vi "Grenzwerte SysLog.vi"(9 "Anlagen-Grenzwerte Anzeige":T1[](array[typedef]) {"Regler" items=["inaktiv", "aktiv"]; "Abschalt-Max" format="%#_5g"; "Abschalt-Min" format="%#_5g"; "Warn-Max" format="%#_5g"; "Warn-Min" format="%#_5g"; "Sollwert" format="%#_5g"}, 10 "Fehlermeldung":string[](array[string]), 11 "NewVal":T1[](array[typedef]) {"Regler" items=["inaktiv", "aktiv"]; "Abschalt-Max" format="%#_5g"; "Abschalt-Min" format="%#_5g"; "Warn-Max" format="%#_5g"; "Warn-Min" format="%#_5g"; "Sollwert" format="%#_5g"}) -> ()   [LabVIEW 2015, in "Anlagengrenzwerte.lvlib"]
uses:
  Anlagengrenzwerte.lvlib
  Anlagen-Parameter Anzeige.ctl
  Visualisierungs Elemente/Zahlen-Eingabefeld.ctl
  SysLog/SysLog Interface.ctl
  SysLog/SysLog.lvlib
panel:
  # "°C"
  # "°C"
  # "°C"
  # "°C"
  # "°C"
  # "°C"
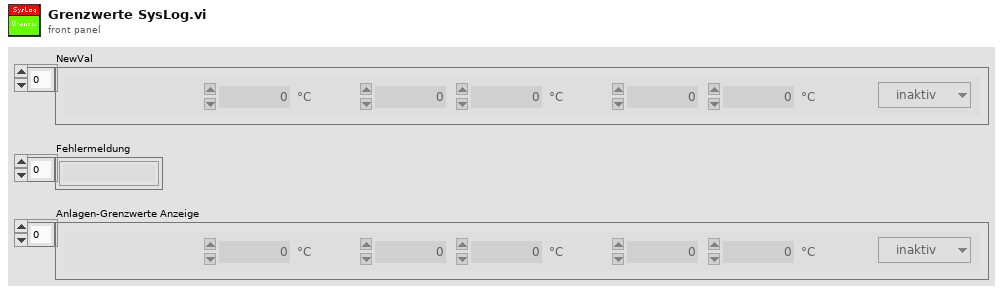
[diagram p1: front panel]
types:
  T1 = typedef "Anlagengrenzwerte.lvlib/Anlagen-Parameter Anzeige.ctl" = cluster{"Sollwert":T2, "Warn-Min":T2, "Warn-Max":T2, "Abschalt-Min":T2, "Abschalt-Max":T2, "Regler":u16}
  T2 = typedef "Zahlen-Eingabefeld.ctl" = sgl
  T3 = typedef "SysLog.lvlib/SysLog Interface.ctl" = cluster{"FehlermeldungsCode":i32, "ErfolgsmeldungsCode":i32, "ParameterListenString":string, "Anzeige":bool, "SysLogIcon":enum16{"OK", "Warnung", "Fehler"}, "intern":bool}
  T4 = cluster{"Sollwert":T2, "Warn-Min":T2, "Warn-Max":T2, "Abschalt-Min":T2, "Abschalt-Max":T2, "Regler":sgl}
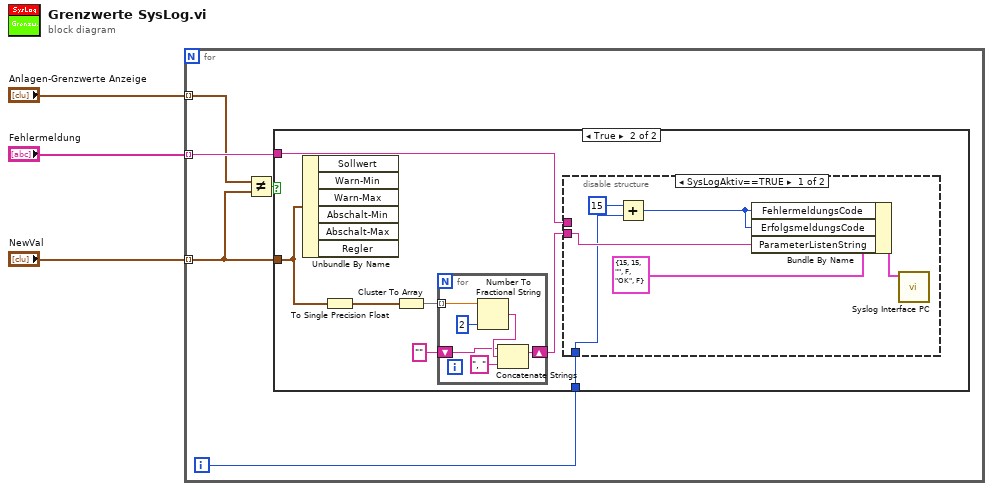
[diagram p0: block diagram]
diagram:
  n1 = for {
    tunnel: "NewVal" -> [w6] mode=indexing
    tunnel: "Anlagen-Grenzwerte Anzeige" -> [w7] mode=indexing
    tunnel: "Fehlermeldung" -> [w8] mode=indexing
    i -> [w4]
    n2 = Not Equal?(x=w7, y=w6) -> (x != y?=w5:bool)
    n3 = case shown="True" w5 {
      tunnel: w8 -> [_ w15]
      tunnel: w6 -> [_ w12]
      tunnel: w4 -> [_ w9]
      frame False {
      }
      frame True {
        n4 = Unbundle By Name(w12) -> ()  [unwired: 6 out]
        n5 = To Single Precision Float(number=w12) -> (single precision float=w10:T4)
        n6 = Cluster To Array(cluster=w10) -> (array=w14:T2[])
        n7 = for {
          tunnel: w14 -> [w21] mode=indexing
          shift-right: [w18] -> w11
          shift-left: "" -> [w19]
          n8 = Number To Fractional String(number=w21, precision (6)=i16 2 ("Genauigkeit (6)")) -> (F-format string=w20:string)  [unwired: 2 in]
          n9 = Concatenate Strings(w19, w20, ", " ("String")) -> (w18:string)
        }
        n10 = disable-structure shown="SysLogAktiv==TRUE" {
          disable-tunnel: w15 -> [_ _]
          disable-tunnel: w11 -> [w26 _]
          disable-tunnel: w9 -> [w24 _]
          frame condition #0 (active) {
            n11 = Add(x=15, y=w24) -> (x+y=w22:i32)
            n12 = Bundle By Name(cluster=T3 {"FehlermeldungsCode"=15, "ErfolgsmeldungsCode"=15, "ParameterListenString"="", "Anzeige"=FALSE, "SysLogIcon"=enum."OK", "intern"=FALSE} ("Cluster (in)"), "FehlermeldungsCode"=w22, "ErfolgsmeldungsCode"=w22, "ParameterListenString"=w26) -> (w25:T3)
            n13 = call "Syslog Interface PC.vi"("Cluster (in)"=w25) -> ()  [unwired: 10 in, 1 out]
          }
          frame condition #1 {
          }
        }
      }
    }
  }
